vi "BRig_dataLC_Cue_First_Count_l1.vi"() -> (2 "output_Cue_First_Count":i32)   [LabVIEW 2014]
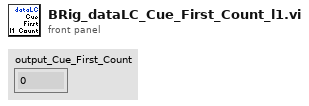
[diagram p1: front panel]
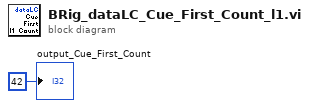
[diagram p0: block diagram]
diagram:
  "output_Cue_First_Count" <- 42 ("output_iBlock")
